vi "ProcessData.vi"(8 "error in (no error)":errorcluster, 9 "State":T1, 10 "Analog Data":T3, 11 "BehaviorClassification in":refnum<class "ClassDiscrimination.lvclass">) -> (0 "error out":errorcluster, 1 "Fixated":bool, 2 "Trigger":T2=enum."Broke Fixation", 3 "BehaviorClassification out":refnum<class "ClassDiscrimination.lvclass">)   [LabVIEW 2014, in "ClassDiscrimination.lvclass"]
uses:
  ClassDiscrimination.lvclass
  Core SubVIs/Controls/TYPE - Analog Data.ctl
  Trial Based Experiment Statechart/Trial Based Experiment.lvsc/Trigger.ctl
  Trial Based Experiment Statechart/Trial Based Experiment.lvsc/State.ctl
  ClassDiscrimination.lvclass/ClassDiscrimination.ctl
  <vilib>/measure/madcrms.llb/Basic Averaged DC-RMS for 1 Chan.vi
  Trial Based Experiment Statechart/Trial Based Experiment.lvsc
  Core SubVIs/Core SubVIs.lvlib
  <vilib>/measure/NI_MAPro.lvlib
  Acquisition/BehaviorData/BehaviorData.lvclass
panel:
  in  "Adjustment Rate":dbl=0.02
  in  "Target Distance":dbl=300.0
  in  "Incorrect":bool
  in  "Correct":bool
  in  "Toggle Fixation":bool
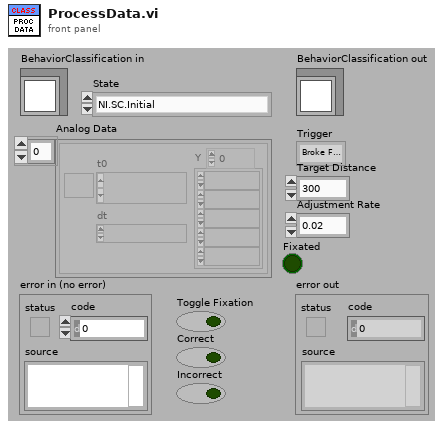
[diagram p1: front panel]
types:
  T1 = typedef "Trial Based Experiment.lvsc/State.ctl" = enum16{"NI.SC.Initial", "NI.SC.History", "NI.SC.ShallowHistory", "NI.SC.Terminal", "Cleanup", "State", "State\\Region\\Pause", "State\\Region\\Response Period", "State\\Region\\Delay Period", "State\\Region\\Hold Fixation", "State\\Region\\Acquire Fixation", "State\\Region\\Abort Trial", "State\\Region\\End Trial", "State\\Region\\Intertrial", "State\\Region\\Start Trial"}
  T2 = typedef "Trial Based Experiment.lvsc/Trigger.ctl" = enum16{"NULL", "Fixated", "Broke Fixation", "Stop", "Correct Response", "Incorrect Response", "Timeout"}
  T3 = typedef "Core SubVIs.lvlib/TYPE - Analog Data.ctl" = waveform(dbl)[]
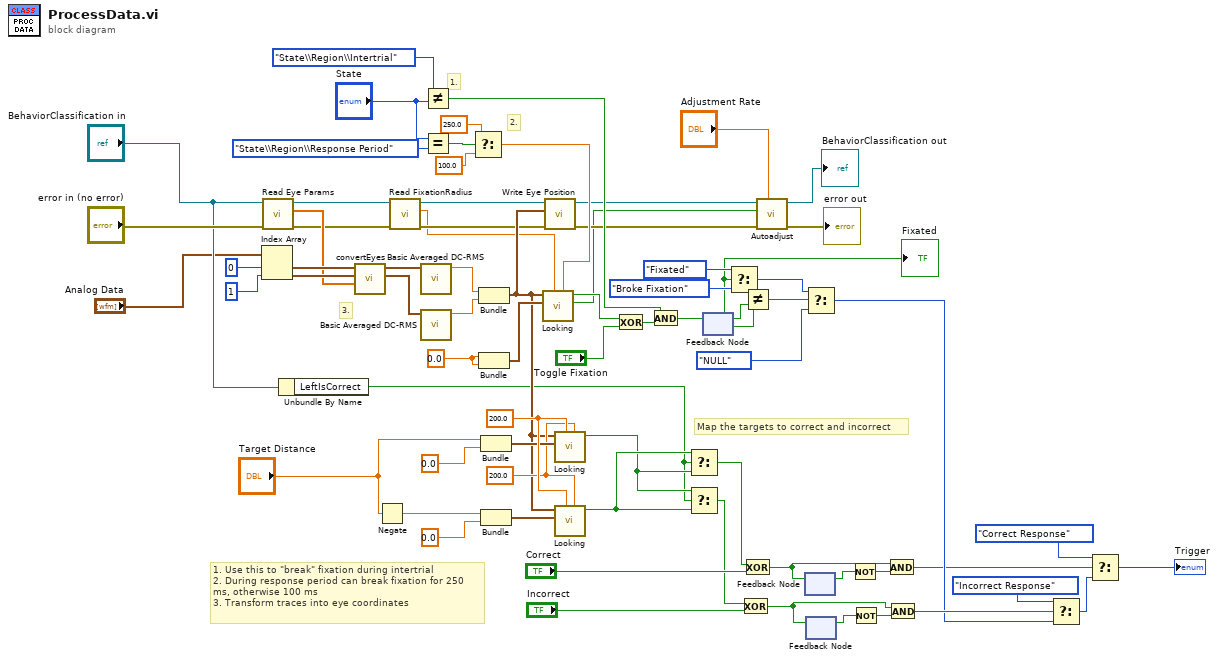
[diagram p0: block diagram]
diagram:
  w33 = 200.0
  w42 = 200.0 ("Fixation Radius (px)")
  w47 = 0.0
  # "3."
  # "1."
  # "2."
  # "1. Use this to \"break\" fixation during intertrial\n2. During response period can break fixation for 250\nms, otherwise 100 ms\n3. Transform traces into eye coordinates"
  # "Map the targets to correct and incorrect"
  n1 = Index Array(array="Analog Data", index #1=0 ("index"), index #2=1 ("index")) -> (element #1=w71:waveform(dbl), element #2=w70:waveform(dbl))
  n2 = call-dynamic "Read Eye Params.vi"("error in (no error)"="error in (no error)", "TrialBasedExperiment in"="BehaviorClassification in") -> ("error out"=w24:errorcluster, "Eye Params"=w62:dbl[], "TrialBasedExperiment out"=w25:refnum<class "ClassDiscrimination.lvclass">)  [unwired: 7 in]
  n3 = Unbundle By Name("BehaviorClassification in") -> ("LeftIsCorrect"=w20:bool)
  n4 = call "convertEyes.vi"("Params"=w62, "Vertical"=w70, "Horizontal"=w71) -> ("Vertical Calibrated"=w68:waveform(dbl), "Horizontal Calibrated"=w69:waveform(dbl))  [unwired: 7 in]
  n5 = Negate(x="Target Distance") -> (-x=w27:dbl)
  n6 = call-dynamic "Read FixationRadius.vi"("error in (no error)"=w24, "MatlabExperiment in"=w25) -> ("error out"=w22:errorcluster, "FixationRadius"=w21:dbl, "MatlabExperiment out"=w23:refnum<class "ClassDiscrimination.lvclass">)  [unwired: 7 in]
  n7 = call-poly <vilib>:"Basic Averaged DC-RMS.vi"("signal in"=w69) -> ("DC value"=w50:dbl)  [unwired: 7 in, 3 out]
  n8 = call-poly <vilib>:"Basic Averaged DC-RMS.vi"("signal in"=w68) -> ("DC value"=w49:dbl)  [unwired: 7 in, 3 out]
  n9 = Not Equal?(x=State."State\\Region\\Intertrial", y="State") -> (x != y?=w17:bool)
  n10 = Equal?(x="State", y=State."State\\Region\\Response Period") -> (x = y?=w14:bool)
  n11 = Select(t=250.0 ("Break Timeout (ms)"), s=w14, f=100.0) -> (s? t:f=w11:dbl)
  n12 = Bundle("DC value"=w50, "DC value"=w49) -> (w26:cluster{"DC value":dbl, "DC value":dbl})  [unwired: 1 in]
  n13 = Bundle(w47, w47) -> (w48:cluster{dbl, dbl})  [unwired: 1 in]
  n14 = Bundle("Target Distance"="Target Distance", 0.0) -> (w40:cluster{"Target Distance":dbl, dbl})  [unwired: 1 in]
  n15 = Bundle(w27, 0.0) -> (w38:cluster{dbl, dbl})  [unwired: 1 in]
  n16 = call "Looking.vi"("Break Timeout (ms)"=w11, "Fixation Radius (px)"=w21, "Desired Position"=w48, "Eye Position"=w26) -> ("Looking Unfiltered"=w2:bool, "Looking"=w45:bool)  [unwired: 6 in]
  n17 = call-dynamic "Write Eye Position.vi"("error in (no error)"=w22, "Eye Position"=w26, "TrialBasedExperiment in"=w23) -> ("error out"=w7:errorcluster, "TrialBasedExperiment out"=w8:refnum<class "ClassDiscrimination.lvclass">)  [unwired: 7 in]
  n18 = call "Looking.vi"("Break Timeout (ms)"=w33, "Fixation Radius (px)"=w42, "Desired Position"=w40, "Eye Position"=w26) -> ("Looking"=w31:bool)  [unwired: 6 in, 1 out]
  n19 = call "Looking.vi"("Break Timeout (ms)"=w33, "Fixation Radius (px)"=w42, "Desired Position"=w38, "Eye Position"=w26) -> ("Looking"=w32:bool)  [unwired: 6 in, 1 out]
  n20 = Exclusive Or(1:"Toggle Fixation", 2:w45) -> (0:w18:bool)
  n21 = And(x=w17, y=w18) -> (x .and. y?=w5:bool)
  "Fixated" <- w5
  n22 = Select(t=w32, s=w20, f=w31) -> (s? t:f=w30:bool)
  n23 = Select(t=w31, s=w20, f=w32) -> (s? t:f=w29:bool)
  n24 = feedback #1() -> (w67:bool)  [unwired: 1 in]
  n25 = feedback-in #1(w5) -> ()
  n26 = Select(t=Trigger."Fixated" ("Trigger"), s=w5, f=Trigger."Broke Fixation" ("Trigger")) -> (s? t:f=w65:T2)
  n27 = Exclusive Or(1:"Incorrect", 2:w29) -> (0:w34:bool)
  n28 = Not Equal?(x=w5, y=w67) -> (x != y?=w9:bool)
  n29 = Exclusive Or(1:"Correct", 2:w30) -> (0:w36:bool)
  n30 = call-dynamic "Autoadjust.vi"("Adjustment Rate"="Adjustment Rate", "error in (no error)"=w7, "Fixated"=w2, "TrialBasedExperiment in"=w8) -> ("error out"=→"error out":errorcluster, "TrialBasedExperiment out"=→"BehaviorClassification out":refnum<class "ClassDiscrimination.lvclass">)  [unwired: 6 in]
  n31 = feedback #2() -> (w60:bool)  [unwired: 1 in]
  n32 = feedback-in #2(w36) -> ()
  n33 = Select(t=w65, s=w9, f=Trigger."NULL" ("Trigger")) -> (s? t:f=w55:T2)
  n34 = feedback #3() -> (w58:bool)  [unwired: 1 in]
  n35 = feedback-in #3(w34) -> ()
  n36 = Not(x=w60) -> (.not. x?=w59:bool)
  n37 = Not(x=w58) -> (.not. x?=w57:bool)
  n38 = And(x=w36, y=w59) -> (x .and. y?=w54:bool)
  n39 = And(x=w34, y=w57) -> (x .and. y?=w56:bool)
  n40 = Select(t=Trigger."Incorrect Response", s=w56, f=w55) -> (s? t:f=w53:T2)
  n41 = Select(t=Trigger."Correct Response", s=w54, f=w53) -> (s? t:f=→"Trigger":T2)
